vi "WAIT_FOR_PID.vi"(10 "argv":string[](array[string]), 11 "args":u8) -> ()   [LabVIEW 2015]
uses:
  Team Code/Robot Global Data.vi
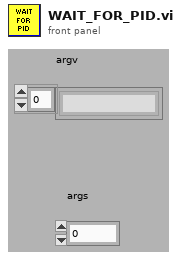
[diagram p1: front panel]
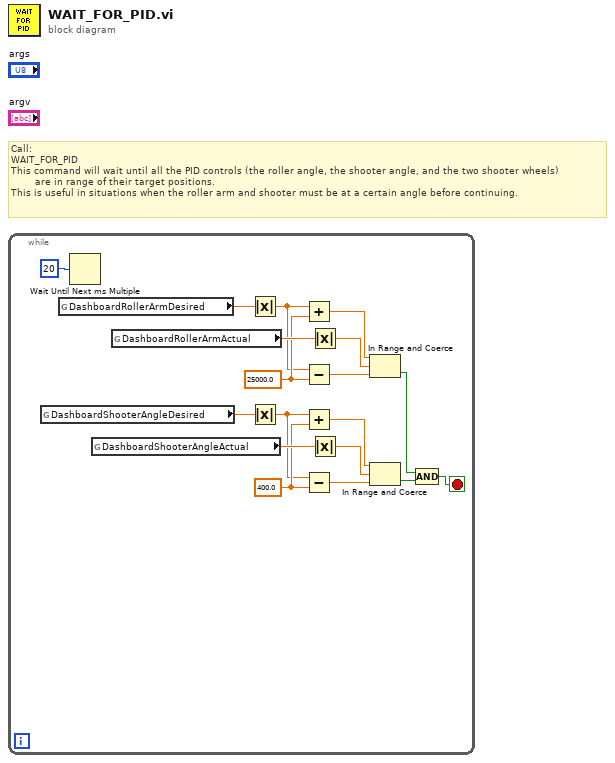
[diagram p0: block diagram]
diagram:
  # "Call:\nWAIT_FOR_PID\nThis command will wait until all the PID controls (the roller angle, the shooter angle, and the two shooter wheels)\n        are in range of their target positions.\nThis is useful in situations when the roller arm and shooter must be at a certain angle before continuing."
  n1 = while {
    stop <- w1 stop-if-true
    w4 = 25000.0 ("y")
    w5 = 400.0 ("y")
    n2 = global read "Robot Global Data.vi" "DashboardShooterAngleDesired"() -> (w11:dbl)
    n3 = global read "Robot Global Data.vi" "DashboardRollerArmDesired"() -> (w15:dbl)
    n4 = Wait Until Next ms Multiple(millisecond multiple=u32 20) -> ()  [unwired: 1 out]
    n5 = global read "Robot Global Data.vi" "DashboardShooterAngleActual"() -> (w14:dbl)
    n6 = global read "Robot Global Data.vi" "DashboardRollerArmActual"() -> (w18:dbl)
    n7 = Absolute Value(x=w15) -> (abs(x)=w3:dbl)
    n8 = Absolute Value(x=w11) -> (abs(x)=w2:dbl)
    n9 = Add(x=w3, y=w4) -> (x+y=w17:dbl)
    n10 = Subtract(x=w3, y=w4) -> (x-y=w16:dbl)
    n11 = Add(x=w2, y=w5) -> (x+y=w13:dbl)
    n12 = Subtract(x=w2, y=w5) -> (x-y=w12:dbl)
    n13 = Absolute Value(x=w18) -> (abs(x)=w6:dbl)
    n14 = Absolute Value(x=w14) -> (abs(x)=w7:dbl)
    n15 = In Range and Coerce(upper limit=w17, x=w6, lower limit=w16) -> (In Range?=w10:bool)  [unwired: 1 out]
    n16 = In Range and Coerce(upper limit=w13, x=w7, lower limit=w12) -> (In Range?=w9:bool)  [unwired: 1 out]
    n17 = Compound Arithmetic op=AND(w10, w9) -> (w1:bool)
  }
